vi "String in Array suchen.vi"(9 "Nach String/Zeichen suchen (-)":string, 11 "String-Array":string[](array[string])) -> (0 "Einheit":string, 1 "Index":i32, 3 "Gefunden?":bool)   [LabVIEW 2020, in "allgemeine Sub-VIs.lvlib"]
uses:
  allgemeine Sub-VIs.lvlib
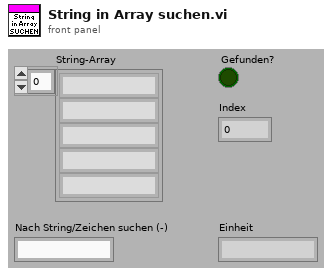
[diagram p1: front panel]
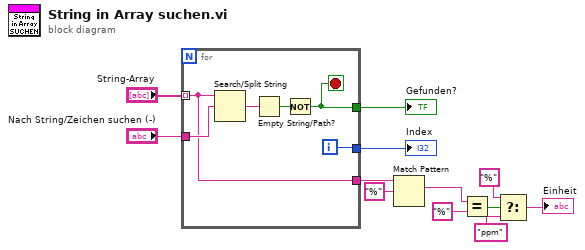
[diagram p0: block diagram]
diagram:
  n1 = for {
    tunnel: "Nach String/Zeichen suchen (-)" -> [w18]
    tunnel: "String-Array" -> [w13] mode=indexing
    tunnel: [w15] -> w9
    tunnel: [w14] -> w10
    tunnel: [w13] -> w3
    i -> [w14]
    stop <- w15 stop-if-true
    n2 = Search/Split String(string=w13, search string/char (-)=w18) -> (match + rest of string=w17:string)  [unwired: 1 in, 2 out]
    n3 = Empty String/Path?(string/path=w17) -> (empty?=w16:bool)
    n4 = Not(x=w16) -> (.not. x?=w15:bool)
  }
  "Index" <- w10
  "Gefunden?" <- w9
  n5 = Match Pattern(string=w3, regular expression="%" ("Regulärer Ausdruck")) -> (match substring=w4:string)  [unwired: 1 in, 3 out]
  n6 = Equal?(x=w4, y="%") -> (x = y?=w7:bool)
  n7 = Select(t="%" ("y"), s=w7, f="ppm") -> (s? t:f=→"Einheit":string)
